vi "Timeout.vi"(8 "Start Time In":u32, 11 "Limit In":u32) -> (0 "Start Time Out":u32, 3 "Timeout":bool)   [LabVIEW 2019]
panel:
  out "Tick counter":u32
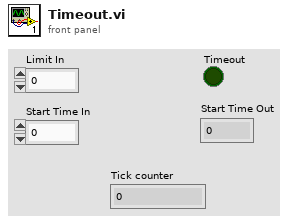
[diagram p1: front panel]
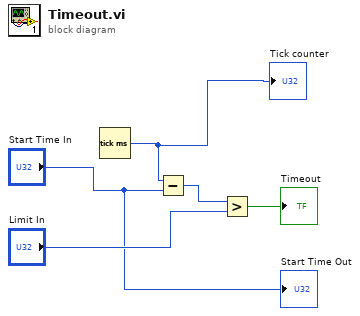
[diagram p0: block diagram]
diagram:
  n1 = Tick Count (ms)() -> (millisecond timer value=w2:u32)
  "Tick counter" <- w2
  n2 = Subtract(x=w2, y="Start Time In") -> (x-y=w5:u32)
  n3 = Greater?(x=w5, y="Limit In") -> (0:→"Timeout":bool)
  "Start Time Out" <- "Start Time In"
